vi "IC Barcode.vi"() -> ()   [LabVIEW 2013]
uses:
  TIS.Imaging.ICImagingControl34
  C:/Program Files (x86)/The Imaging Source Europe GmbH/IC Barcode/TIS.Imaging.Barcode.dll
  Program Files (x86)/The Imaging Source Europe GmbH/IC Barcode/TIS.Imaging.Barcode.dll
panel:
  out "Barcode":string
  in  "stop":bool
  in  "ICImagingControl":refnum<k24>(container)
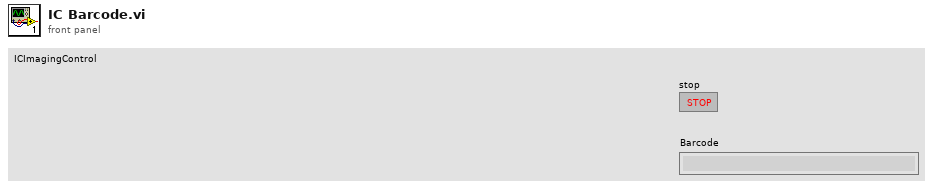
[diagram p1: front panel]
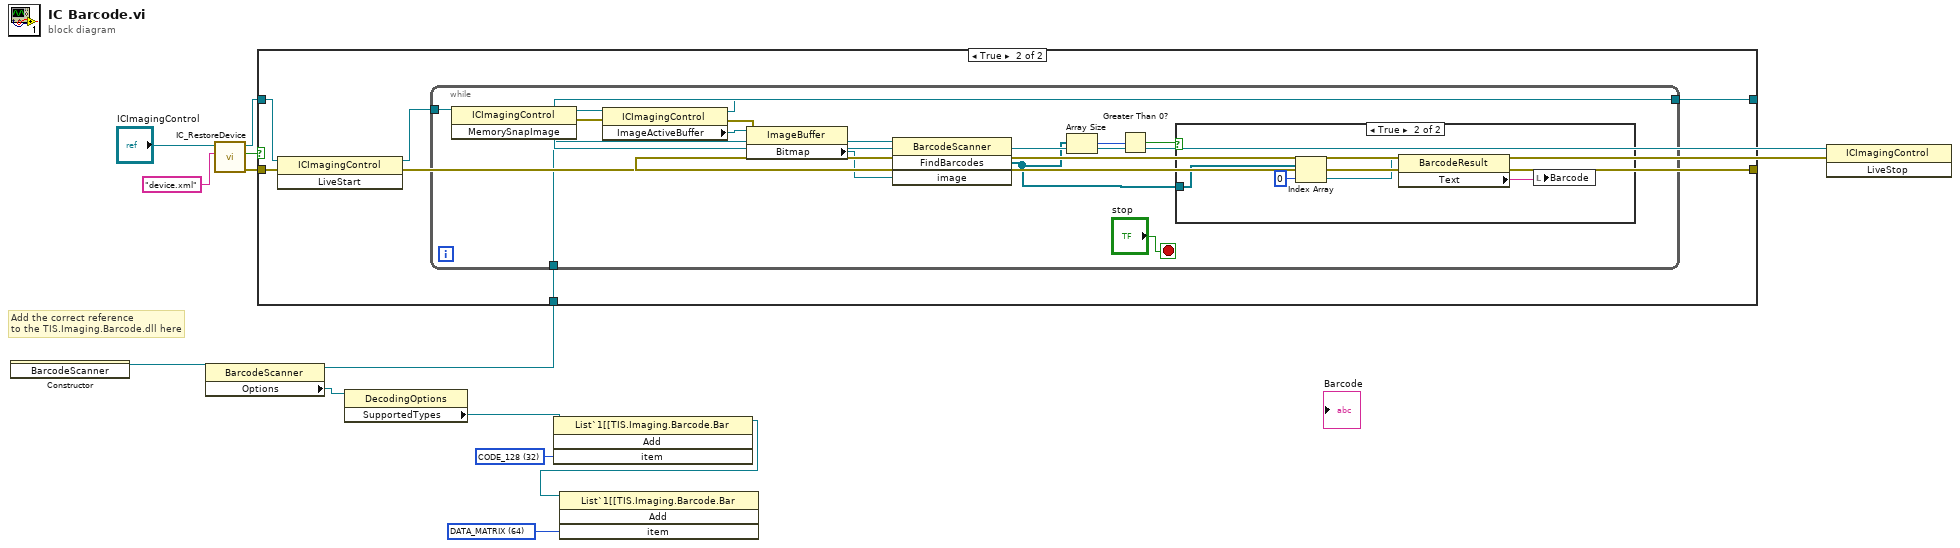
[diagram p0: block diagram]
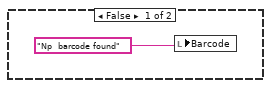
[diagram p3: hidden frame]
diagram:
  w2 = 64 items=["AZTEC"=2, "CODE_39"=8, "CODE_93"=16, "CODE_128"=32, "DATA_MATRIX"=64, "EAN_8"=128, "EAN_13"=256, "MAXICODE"=1024, "PDF_417"=2048, "QR_CODE"=4096, "UPC_A"=32768, "UPC_E"=65536, "UPC_EAN_EXTENSION"=131072, "INTERLEAVED_2_OF_5"=262144] ("item")
  w4 = 32 items=["AZTEC"=2, "CODE_39"=8, "CODE_93"=16, "CODE_128"=32, "DATA_MATRIX"=64, "EAN_8"=128, "EAN_13"=256, "MAXICODE"=1024, "PDF_417"=2048, "QR_CODE"=4096, "UPC_A"=32768, "UPC_E"=65536, "UPC_EAN_EXTENSION"=131072, "INTERLEAVED_2_OF_5"=262144] ("item")
  # "Add the correct reference \nto the TIS.Imaging.Barcode.dll here"
  n1 = constructor class="BarcodeScanner"() -> (reference out=w7:refnum<k24>)  [unwired: 3 in, 2 out]
  n2 = property class="BarcodeScanner"(reference=w7) -> (reference out=w1:refnum<k24>, "Options"=w6:refnum<k24>)  [unwired: 1 in, 1 out]
  n3 = call "IC_RestoreDevice.vi"("filename"="device.xml", ".NET Refnum in"="ICImagingControl") -> ("error out"=w9:errorcluster, "DeviceValid"=w8:bool, ".NET Refnum out"=w10:refnum<k24>)  [unwired: 7 in]
  n4 = case shown="True" w8 {
    tunnel: [w16 w17] -> w14
    tunnel: [w15 w21] -> w13
    tunnel: w10 -> [w16 w20]
    tunnel: w9 -> [w15 w19]
    tunnel: w1 -> [_ w18]
    frame False {
    }
    frame True {
      n5 = invoke class="ICImagingControl" method="LiveStart"(reference=w20, error in=w19) -> (reference out=w22:refnum<k24>, error out=w21:errorcluster)  [unwired: 1 in, 1 out]
      n6 = while {
        tunnel: w22 -> [w33]
        tunnel: w18 -> [w28]
        tunnel: [w26] -> w17
        stop <- "stop" stop-if-true
        n7 = invoke class="ICImagingControl" method="MemorySnapImage"(reference=w33) -> (reference out=w32:refnum<k24>, error out=w31:errorcluster)  [unwired: 2 in, 1 out]
        n8 = property class="ICImagingControl"(reference=w32, error in=w31) -> (reference out=w26:refnum<k24>, error out=w30:errorcluster, "ImageActiveBuffer"=w29:refnum<k24>)
        n9 = property class="ImageBuffer"(reference=w29, error in=w30) -> ("Bitmap"=w27:refnum<k24>)  [unwired: 2 out]
        n10 = invoke class="BarcodeScanner" method="FindBarcodes"(reference=w28, "image"=w27) -> ("FindBarcodes"=w25:refnum<k24>[])  [unwired: 2 in, 3 out]
        n11 = Array Size(array=w25) -> (size(s)=w24:i32)
        n12 = Greater Than 0?(x=w24) -> (x > 0?=w23:bool)
        n13 = case shown="True" w23 {
          tunnel: w25 -> [_ w37]
          frame False {
            n14 = local write "Barcode"("Np  barcode found" ("Text 2")) -> ()
          }
          frame True {
            n15 = Index Array(array=w37, index=0) -> (element=w38:refnum<k24>)
            n16 = property class="BarcodeResult"(reference=w38) -> ("Text"=w36:string)  [unwired: 1 in, 2 out]
            n17 = local write "Barcode"(w36) -> ()
          }
        }
      }
    }
  }
  n18 = property class="DecodingOptions"(reference=w6) -> ("SupportedTypes"=w5:refnum<k24>)  [unwired: 1 in, 2 out]
  n19 = invoke class="List`1[[TIS.Imaging.Barcode.Bar" method="Add"(reference=w5, "item"=w4) -> (reference out=w3:refnum<k24>)  [unwired: 2 in, 3 out]
  n20 = invoke class="List`1[[TIS.Imaging.Barcode.Bar" method="Add"(reference=w3, "item"=w2) -> ()  [unwired: 2 in, 4 out]
  n21 = invoke class="ICImagingControl" method="LiveStop"(reference=w14, error in=w13) -> ()  [unwired: 1 in, 3 out]
